vi "Configure Multi Eval Meas Limit ACLR.vi"(4 "Absolute Level (0.0)":dbl format="%^.3e", 5 "Absolute Level Enabled (Off)":i32(ring) items=["Off", "On", "Value"], 6 "Relative Level (0.0)":dbl format="%^.3e", 7 "Relative Level Enabled (Value)":i32(ring)=2 items=["Off", "On", "Value"], 8 "error in (no error)":errorcluster, 9 "Bandwidth (5 MHz)":T1=5 items=["5 MHz"=5, "10 MHz"=10, "15 MHz"=15, "20 MHz"=20, "25 MHz"=25, "30 MHz"=30, "40 MHz"=40, "50 MHz"=50, "60 MHz"=60, "80 MHz"=80, "90 MHz"=90, "100 MHz"=100], 10 "Instance (1)":T2=1, 11 "VISA resource name":refnum<visa-resource-name>) -> (0 "error out":errorcluster, 3 "VISA resource name out":refnum<visa-resource-name>)   [LabVIEW 2020, in "Rohde&Schwarz CMWXP NR FR1 Measurement.lvlib"]
doc: "Defines relative and absolute limits for the ACLR measured in an adjacent NR channel (for NR SA). The settings are defined separately for each channel bandwidth.\n\nAttribute:\nRSCMWXPNRFR1M_ATTR_MULTI_EVAL_MEAS_LIMIT_ACLR\n\nRemote-control command:\nCONFigure:NRSub:MEAS<i>:MEValuation:LIMit:ACLR:NR:CBANdwidth<bw>"
uses:
  <instrlib>/Rohde&Schwarz CMWXP NR FR1 Measurement/Rohde&Schwarz CMWXP NR FR1 Measurement.lvlib
  <instrlib>/Rohde&Schwarz CMWXP NR FR1 Measurement/Private/_Instance.ctl
  <instrlib>/Rohde&Schwarz CMWXP NR FR1 Measurement/Private/_Bandwidth.ctl
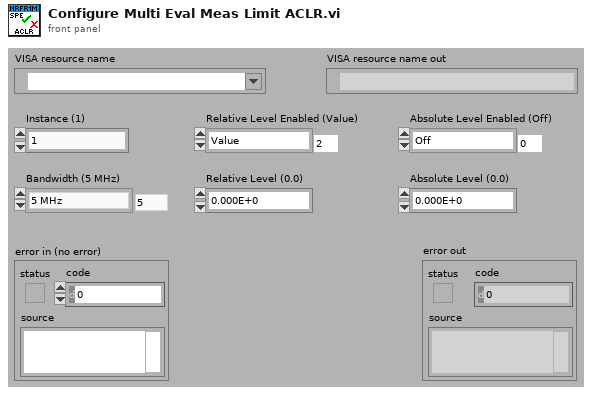
[diagram p1: front panel]
types:
  T1 = typedef "Rohde&Schwarz CMWXP NR FR1 Measurement.lvlib/_Bandwidth.ctl" = i32
  T2 = typedef "Rohde&Schwarz CMWXP NR FR1 Measurement.lvlib/_Instance.ctl" = i32
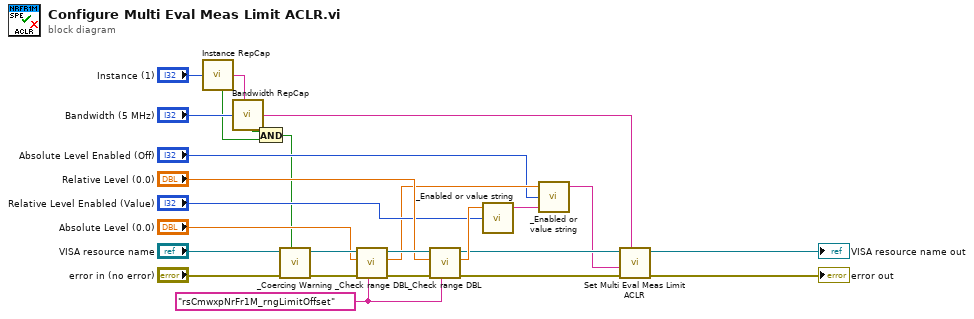
[diagram p0: block diagram]
diagram:
  w16 = "rsCmwxpNrFr1M_rngLimitOffset" ("Range Table Identifier")
  n1 = call <instrlib>:"Instance RepCap.vi"("Instance In"="Instance (1)") -> ("In Range?"=w3:bool, "RepCap Identifier Out"=w6:string)  [unwired: 1 in]
  n2 = call <instrlib>:"Bandwidth RepCap.vi"("Bandwidth (5 MHz)"="Bandwidth (5 MHz)", "RepCap String In (\"\")"=w6) -> ("In Range?"=w2:bool, "RepCap Identifier Out"=w8:string)
  n3 = And(x=w2, y=w3) -> (x .and. y?=w1:bool)
  n4 = call <instrlib>:"_Coercing Warning.vi"("In Range?"=w1, "error in (no error)"="error in (no error)", "VISA resource name"="VISA resource name") -> ("error out"=w21:errorcluster, "VISA resource name out"=w20:refnum<visa-resource-name>)  [unwired: 7 in]
  n5 = call <instrlib>:"_Check range DBL.vi"("Range Table Identifier"=w16, "error in (no error)"=w21, "DBL Value In"="Absolute Level (0.0)", "VISA resource name"=w20) -> ("error out"=w18:errorcluster, "DBL Value Out"=w12:dbl, "VISA resource name out"=w17:refnum<visa-resource-name>)  [unwired: 5 in]
  n6 = call <instrlib>:"_Check range DBL.vi"("Range Table Identifier"=w16, "error in (no error)"=w18, "DBL Value In"="Relative Level (0.0)", "VISA resource name"=w17) -> ("error out"=w10:errorcluster, "DBL Value Out"=w14:dbl, "VISA resource name out"=w9:refnum<visa-resource-name>)  [unwired: 5 in]
  n7 = call <instrlib>:"_Enabled or value string.vi"("Enabled or Value"="Relative Level Enabled (Value)", "Value"=w14) -> ("Resulting String"=w4:string)  [unwired: 3 in]
  n8 = call <instrlib>:"_Enabled or value string.vi"("Initial String"=w4, "Enabled or Value"="Absolute Level Enabled (Off)", "Value"=w12) -> ("Resulting String"=w5:string)  [unwired: 2 in]
  n9 = call "Set Multi Eval Meas Limit ACLR"("Repeated Capabilities"=w8, "error in (no error)"=w10, "Multi Eval Meas Limit ACLR ()"=w5, "instrument handle"=w9) -> ("error out"=→"error out":errorcluster, "instrument handle out"=→"VISA resource name out":refnum<visa-resource-name>)  [unwired: 6 in]
